vi "Pre Launch Init.vi"(11 "Database_handler in":refnum<class "Database_handler.lvclass">) -> (0 "error out":errorcluster, 3 "Database_handler out":refnum<class "Database_handler.lvclass">)   [LabVIEW 2025, in "Database_handler.lvlib" / "Database_handler.lvclass"]
doc: "<p>(<strong>Filename</strong>: <span class=\"dnl\">Actor Framework.lvlib:Actor.lvclass:Pre Launch Init.vi</span>)</p>\n<p>Defines behavior that occurs after the <a href=\"nihelplauncher://docs/csh?context=lvcore_lvcomm_af_launch_nested_actor\">Launch Nested Actor</a> method is invoked but before the actor's Actor Core method begins running.</p>\n<p>By default, this method does nothing. A descendant class may override it to define behavior.</p>"
uses:
  Database_handler.lvclass
  Database_handler.lvclass/Database_handler.ctl
  <vilib>/ActorFramework/Actor/Actor.lvclass
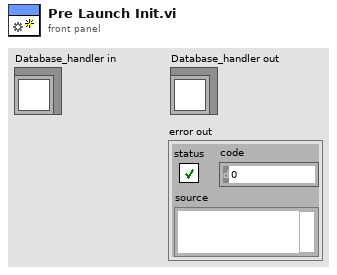
[diagram p1: front panel]
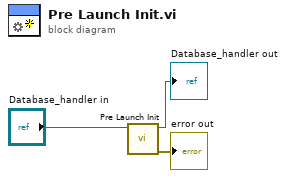
[diagram p0: block diagram]
diagram:
  n1 = call-parent "Pre Launch Init.vi"("Actor in"="Database_handler in") -> ("error out"=→"error out":errorcluster, "Actor out"=→"Database_handler out":refnum<class "Database_handler.lvclass">)  [unwired: 9 in]
